vi "04_error_handler.vi"() -> ()   [LabVIEW 2017]
panel:
  out "error out":errorcluster
  in  "text":string
  in  "file path (use dialog)":path
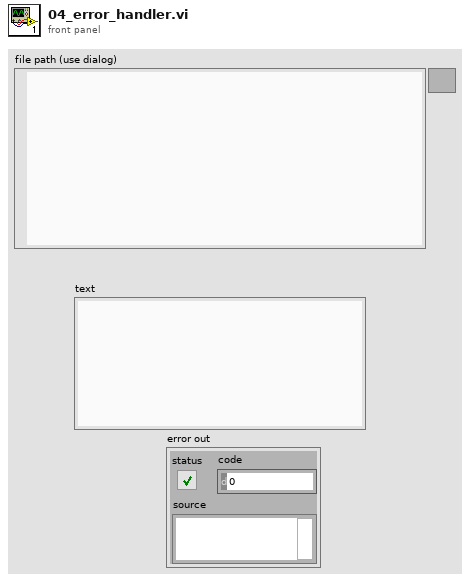
[diagram p1: front panel]
types:
  T1 = enum16{"open", "replace", "create", "open or create", "replace or create", "replace or create with confirmation"}
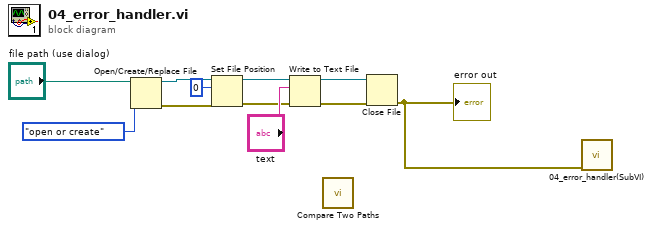
[diagram p0: block diagram]
diagram:
  n1 = Open/Create/Replace File(file path (use dialog)="file path (use dialog)", operation (0:open)=T1."open or create") -> (refnum out=w9:refnum<file>, error out=w4:errorcluster)  [unwired: 4 in, 1 out]
  n2 = Set File Position(offset (in bytes) (0)=i64 0, refnum=w9, error in=w4) -> (refnum out=w8:refnum<file>, error out=w3:errorcluster)  [unwired: 1 in]
  n3 = Write to Text File(file (use dialog)=w8, text="text", error in=w3) -> (refnum out=w7:refnum<file>, error out=w2:errorcluster)  [unwired: 1 in, 1 out]
  n4 = call <vilib>:"Compare Two Paths.vi"() -> ()  [unwired: 8 in, 4 out]
  n5 = Close File(refnum=w7, error in=w2) -> (error out=w1:errorcluster)  [unwired: 1 out]
  "error out" <- w1
  n6 = call "04_error_handler(SubVI).vi"("error in (no error)"=w1) -> ()  [unwired: 11 in]
